vi "Get - Names and Units.vi"(0 "reference in":refnum<class "GSwFormDSP.lvclass">, 5 "error in (no error)":errorcluster) -> (9 "dT Units":string[](array[string]), 11 "Signal Units":string[](array[string]), 13 "Signal Names":string[](array[string]), 14 "reference out":refnum<class "GSwFormDSP.lvclass">, 19 "error out":errorcluster)   [LabVIEW 2020, in "GSwFormDSP.lvclass"]
uses:
  GSwFormDSP.lvclass
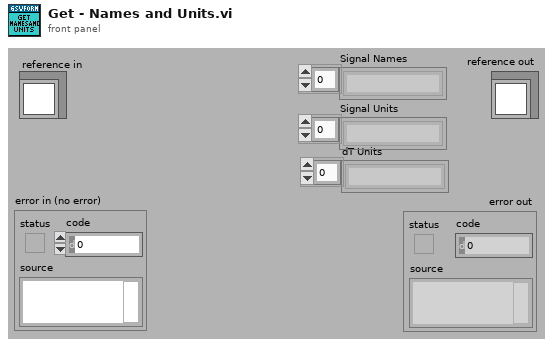
[diagram p1: front panel]
types:
  T1 = typedef "GSwFormDSP.lvclass/ObjectAttributes.ctl" = cluster{"Wform Ref":refnum<data-value>, "Nb Signals":i32, "Spectral Function Parameters":T2, "FFT":waveform(cdb)[], "Nb FFT":i32, "Nb Averages":i32[], "Reference Indexes":i32[], "Response Indexes":i32[], "Coherence":waveform(dbl)[], "TDF Parameters":T4, "DAQ":cluster{"Duration (sec)":dbl, "Buffer Size (Samples)":i32, "Offset (Samples)":i32}, "Filter Impulse Response (TDF)":waveform(dbl), "Sound Playback":T5}
  T2 = typedef "GSwFormDSP.lvclass/Spectral Parameters.ctl" = cluster{"Frequency resolution (Hz)":dbl, "Overlap":dbl, "Window":T3}
  T3 = typedef "NI_AALPro.lvlib/windowTd.ctl" = u32
  T4 = typedef "GSwFormDSP.lvclass/TDF Parameters.ctl" = cluster{"Filter":enum32{"Lowpass", "Highpass", "Bandpass", "Bandstop"}, "Type:":enum16{"Butterworth", "Chebyshev", "Inv Chebyshev", "Elliptic", "Bessel"}, "LP cutoff freq":dbl, "HP cutoff freq":dbl, "Order":i32, "passband ripple (dB)":dbl, "stopband attenuation (dB)":dbl, "Phaseless Filter":bool, "Include Fade IN and OUT":bool}
  T5 = typedef "GSwFormDSP.lvclass/Sound Playback.ctl" = cluster{"Timer start (ms)":u32, "task ID":T6, "Cursor Init Location (s)":dbl, "SC Volume":dbl}
  T6 = typedef "Sound Output Task ID.ctl" = u32
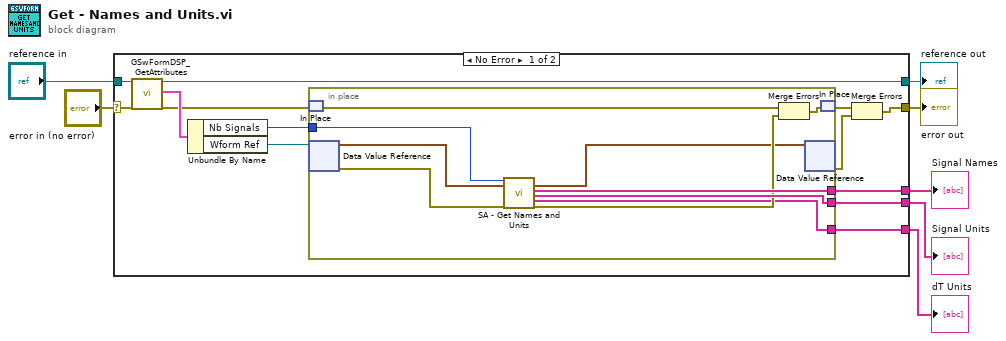
[diagram p0: block diagram]
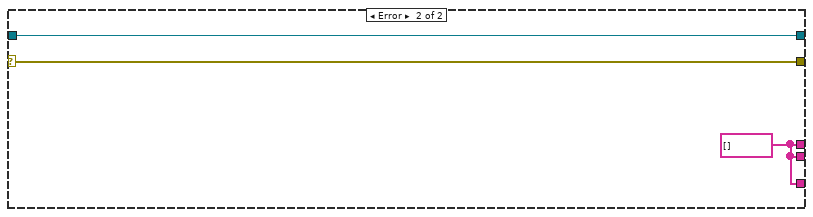
[diagram p2: hidden frame]
diagram:
  n1 = case shown="No Error" "error in (no error)" {
    selector: "error in (no error)" -> [w20 w33]
    tunnel: [w9 w33] -> w6
    tunnel: [w19 w32] -> w4
    tunnel: "reference in" -> [w18 w32]
    tunnel: [w15 w31] -> w3
    tunnel: [w14 w31] -> w2
    tunnel: [w13 w31] -> w1
    frame No Error {
      n2 = call "GSwFormDSP_GetAttributes.vi"("reference in"=w18, "error in (no error)"=w20) -> ("reference out"=w19:refnum<class "GSwFormDSP.lvclass">, "attributes"=w17:T1, "error out"=w12:errorcluster)  [unwired: 14 in, 1 out]
      n3 = Unbundle By Name(w17) -> ("Nb Signals"=w8:i32, "Wform Ref"=w16:refnum<data-value>)
      n4 = in-place {
        in-place-border: [w30] -> w15
        in-place-border: [w29] -> w14
        in-place-border: [w21] -> w13
        in-place-border: w8 -> [w24]
        n5 = in-place-match #1(w12) -> (w28:errorcluster)
        n6 = in-place-dvr #2(w16) -> (w23:waveform(dbl)[], w26:errorcluster)
        n7 = call "SA - Get Names and Units.vi"("Nb Signals"=w24, "Signal IN"=w23, "error in (no error)"=w26) -> ("Signal IN"=w22:waveform(dbl)[], "Signal Names"=w30:string[], "Signal Units"=w29:string[], "dT Units"=w21:string[], "error out"=w25:errorcluster)  [unwired: 12 in]
        n8 = Merge Errors(w28, w25) -> (w27:errorcluster)
        n9 = in-place-dvr #2(w22) -> (w10:errorcluster)  [unwired: 1 out]
        n10 = in-place-match #1(w27) -> (w11:errorcluster)
      }
      n11 = Merge Errors(w11, w10) -> (w9:errorcluster)
    }
    frame Error {
      w31 = string[] []
    }
  }
  "error out" <- w6
  "reference out" <- w4
  "Signal Names" <- w3
  "Signal Units" <- w2
  "dT Units" <- w1
